vi "Auto Near Switch.vi"(10 "Right?":bool) -> ()   [LabVIEW 2017]
uses:
  Auto switch direita.ctl
  LabVIEW_is_Under_Control.lib/Util/Unpack Gamepad/Button Cluster.ctl
  Team Code/Robot Global Data.vi
panel:
  in  "90_time_limit":dbl=1800.0
  in  "Time_limit_fwd_2":dbl=1500.0 format="%#_13g"
  in  "Time_Limit_fwd":dbl=4000.0 format="%#_13g"
  in  "Delay fwd 2":i32=10
  in  "DistanceAfterTurn":dbl=40.0
  in  "Delay Turn":i32=150
  in  "Turn":dbl=-90.0 format="%#_13g"
  in  "Time to wait (min 50ms)":dbl=50.0
  in  "Delay Fwd":i32=100
  in  "DistanceSwitch":dbl=400.0
  out "auto state":T1=enum."Girando"
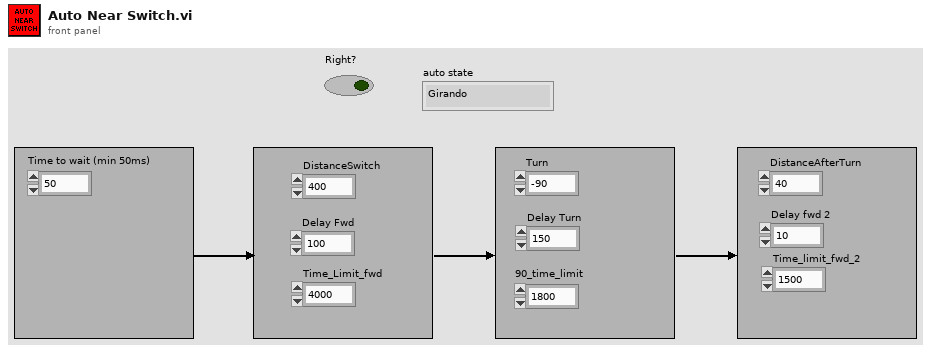
[diagram p1: front panel]
types:
  T1 = typedef "Auto switch direita.ctl" = enum16{"Zerandosensor", "Girando", "Andando", "Jogando", "Andando2", "Finalizando", "Zerandosensor2"}
  T2 = typedef "Button Cluster.ctl" = cluster{"Buttons[0]":bool, "Buttons[1]":bool, "Buttons[2]":bool, "Buttons[3]":bool, "Buttons[4]":bool, "Buttons[5]":bool, "Buttons[6]":bool, "Buttons[7]":bool, "Buttons[8]":bool, "Buttons[9]":bool}
  T3 = cluster{"proportional gain (Kc)":dbl, "integral time (Ti, min)":dbl, "derivative time (Td, min)":dbl}
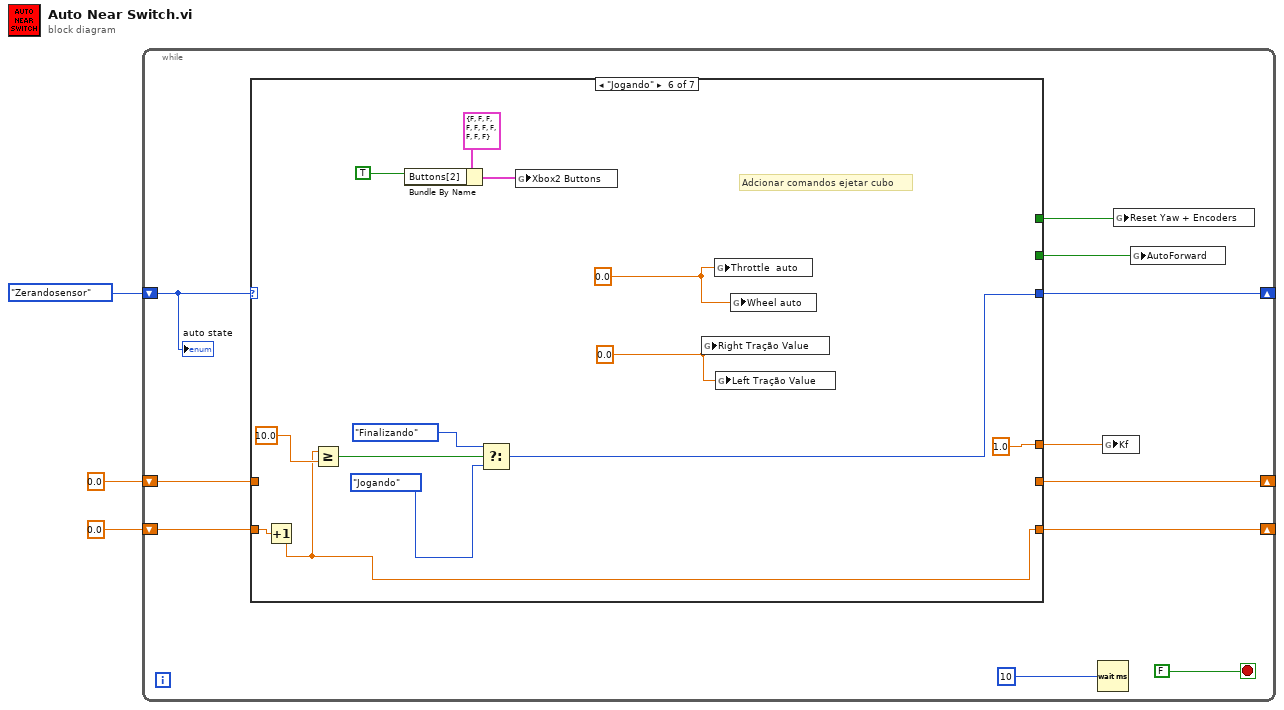
[diagram p0: block diagram]
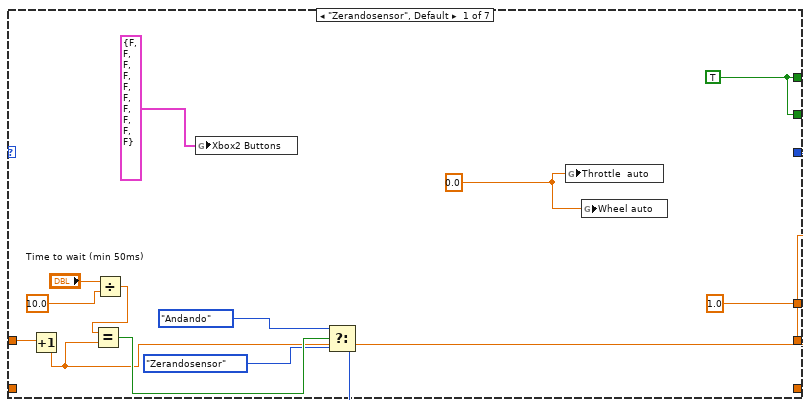
[diagram p2: hidden frame]
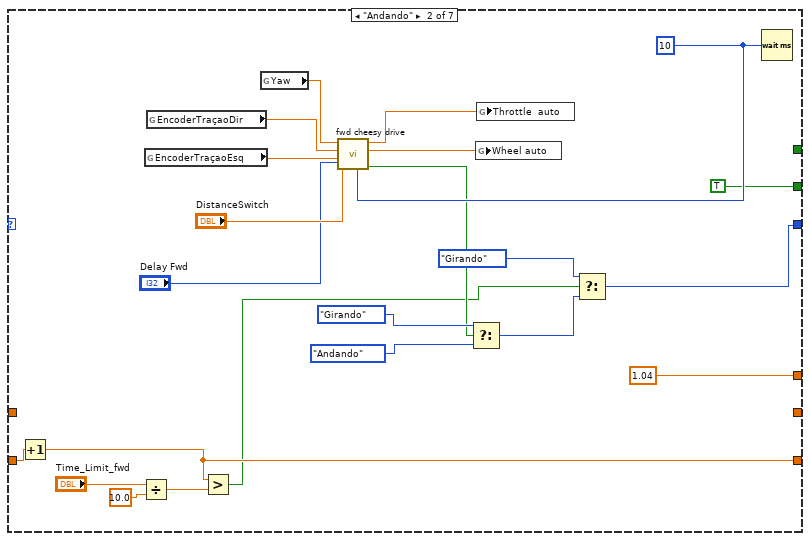
[diagram p3: hidden frame]
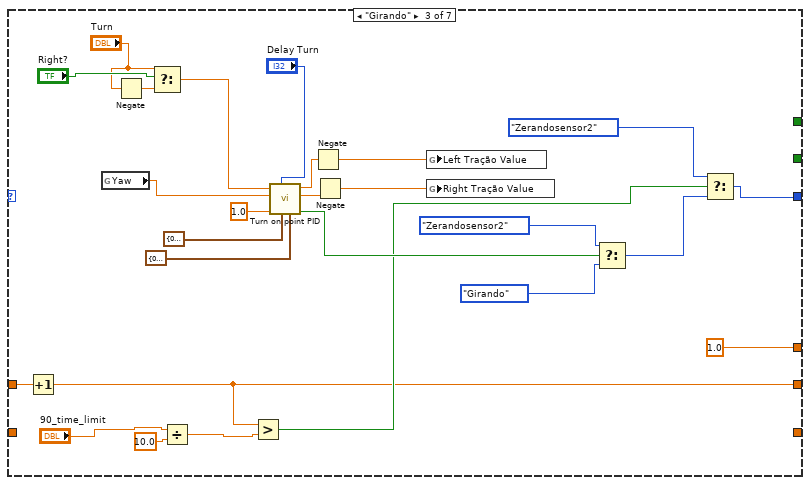
[diagram p4: hidden frame]
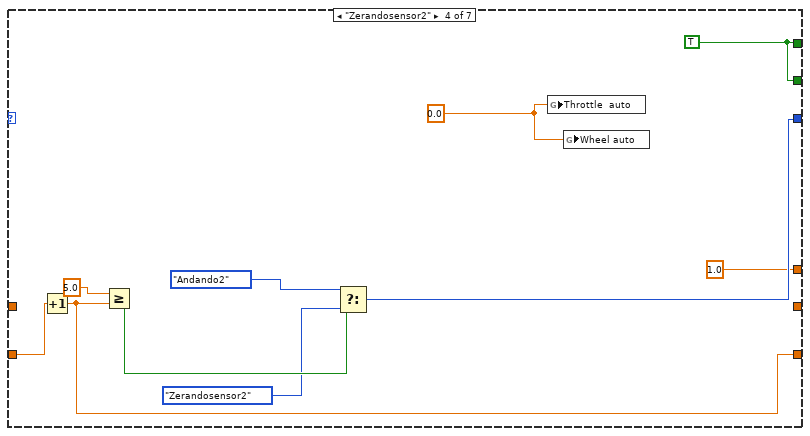
[diagram p5: hidden frame]
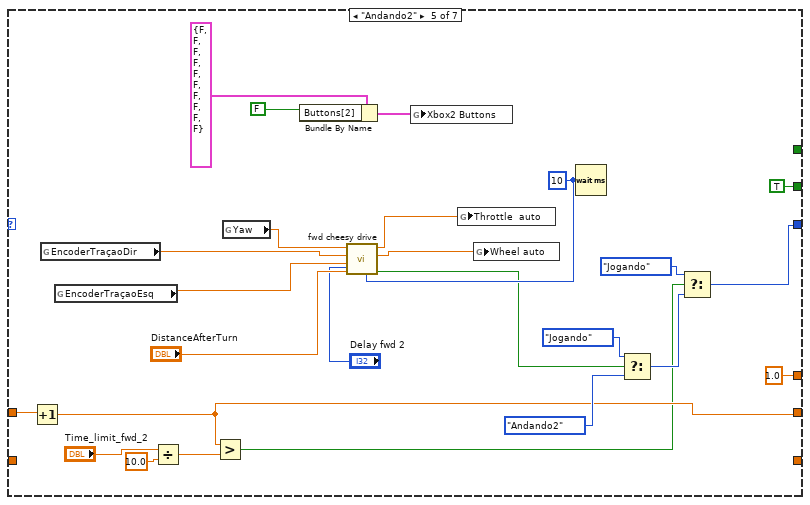
[diagram p6: hidden frame]
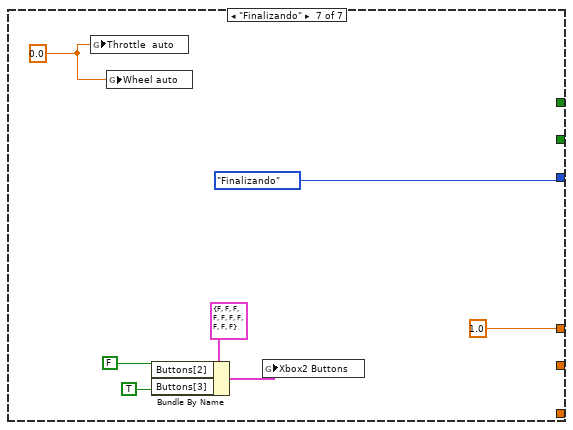
[diagram p7: hidden frame]
diagram:
  n1 = while {
    shift-right: [w10] -> _
    shift-left: Auto_switch_direita."Zerandosensor" -> [w8]
    shift-right: [w11] -> _
    shift-left: 0.0 -> [w12]
    shift-right: [w4] -> _
    shift-left: 0.0 -> [w5]
    stop <- FALSE stop-if-true
    n2 = case shown="\"Jogando\"" w8 {
      tunnel: w12 -> [w16 _ w53 _ w96 _ _]
      tunnel: [w26 _ w52 _ w95 _ _] -> w11
      tunnel: [w25 w35 w55 w79 w91 w122 Auto_switch_direita."Finalizando"] -> w10
      tunnel: [w22 _ _ w84 _ _ _] -> w7
      tunnel: [w22 TRUE _ w84 TRUE _ _] -> w9
      tunnel: [1.0 1.04 1.0 1.0 1.0 1.0 1.0] -> w6
      tunnel: w5 -> [_ w31 _ w77 _ w118 _]
      tunnel: [_ w30 _ w76 _ w111 _] -> w4
      frame "Zerandosensor", Default {
        w21 = 0.0
        w22 = TRUE
        n3 = Increment(x=w16) -> (x+1=w26:dbl)
        n4 = Divide(x="Time to wait (min 50ms)", y=10.0) -> (x/y=w17:dbl)
        n5 = Equal?(x=w17, y=w26) -> (x = y?=w27:bool)
        n6 = global write "Robot Global Data.vi" "Xbox2 Buttons"(T2 {"Buttons[0]"=FALSE, "Buttons[1]"=FALSE, "Buttons[2]"=FALSE, "Buttons[3]"=FALSE, "Buttons[4]"=FALSE, "Buttons[5]"=FALSE, "Buttons[6]"=FALSE, "Buttons[7]"=FALSE, "Buttons[8]"=FALSE, "Buttons[9]"=FALSE} ("Madcatz Buttons")) -> ()
        n7 = Select(t=Auto_switch_direita."Andando", s=w27, f=Auto_switch_direita."Zerandosensor") -> (s? t:f=w25:T1)
        n8 = global write "Robot Global Data.vi" "Throttle  auto"(w21) -> ()
        n9 = global write "Robot Global Data.vi" "Wheel auto"(w21) -> ()
      }
      frame "Andando" {
        w45 = u32 10 ("milliseconds to wait")
        n10 = Increment(x=w31) -> (x+1=w30:dbl)
        n11 = Divide(x="Time_Limit_fwd", y=10.0) -> (x/y=w32:dbl)
        n12 = global read "Robot Global Data.vi" "EncoderTraçaoEsq"() -> (w48:dbl)
        n13 = global read "Robot Global Data.vi" "EncoderTraçaoDir"() -> (w47:dbl)
        n14 = Greater?(x=w30, y=w32) -> (0:w28:bool)
        n15 = global read "Robot Global Data.vi" "Yaw"() -> (w49:dbl)
        n16 = call "fwd cheesy drive.vi"("Loop Timer"=w45, "Time to stop"="Delay Fwd", "Distance"="DistanceSwitch", "Encoder Left"=w48, "Encoder Right"=w47, "Yaw"=w49) -> ("Finished distance"=w29:bool, "Direction"=w43:dbl, "Trottle"=w42:dbl)  [unwired: 2 in, 1 out]
        n17 = Select(t=Auto_switch_direita."Girando", s=w29, f=Auto_switch_direita."Andando") -> (s? t:f=w36:T1)
        n18 = global write "Robot Global Data.vi" "Wheel auto"(w43) -> ()
        n19 = global write "Robot Global Data.vi" "Throttle  auto"(w42) -> ()
        n20 = Select(t=Auto_switch_direita."Girando", s=w28, f=w36) -> (s? t:f=w35:T1)
        n21 = Wait (ms)(milliseconds to wait=w45) -> ()  [unwired: 1 out]
      }
      frame "Girando" {
        n22 = Increment(x=w53) -> (x+1=w52:dbl)
        n23 = global read "Robot Global Data.vi" "Yaw"() -> (w68:dbl)
        n24 = Negate(x="Turn") -> (-x=w63:dbl)
        n25 = Select(t="Turn", s="Right?", f=w63) -> (s? t:f=w61:dbl)
        n26 = Divide(x="90_time_limit", y=10.0) -> (x/y=w59:dbl)
        n27 = Greater?(x=w52, y=w59) -> (0:w57:bool)
        n28 = call "Turn on point PID.vi"("Range"=cluster{"output high":dbl, "output low":dbl} {"output high"=0.65, "output low"=-0.65}, "Gains"=T3 {"proportional gain (Kc)"=0.015, "integral time (Ti, min)"=0.01, "derivative time (Td, min)"=0.0}, "Time to stop"="Delay Turn", "Precision"=1.0, "Yaw"=w68, "Setpoint(degrees)"=w61) -> ("Finished?"=w74:bool, "PWM right"=w70:dbl, "PWM left"=w71:dbl)  [unwired: 3 in]
        n29 = Negate(x=w71) -> (-x=w67:dbl)
        n30 = Negate(x=w70) -> (-x=w66:dbl)
        n31 = global write "Robot Global Data.vi" "Left Tração Value"(w67) -> ()
        n32 = global write "Robot Global Data.vi" "Right Tração Value"(w66) -> ()
        n33 = Select(t=Auto_switch_direita."Zerandosensor2", s=w74, f=Auto_switch_direita."Girando") -> (s? t:f=w56:T1)
        n34 = Select(t=Auto_switch_direita."Zerandosensor2", s=w57, f=w56) -> (s? t:f=w55:T1)
      }
      frame "Zerandosensor2" {
        w84 = TRUE
        w85 = 0.0
        n35 = Increment(x=w77) -> (x+1=w76:dbl)
        n36 = Greater Or Equal?(x=5.0, y=w76) -> (x >= y?=w82:bool)
        n37 = Select(t=Auto_switch_direita."Andando2", s=w82, f=Auto_switch_direita."Zerandosensor2") -> (s? t:f=w79:T1)
        n38 = global write "Robot Global Data.vi" "Throttle  auto"(w85) -> ()
        n39 = global write "Robot Global Data.vi" "Wheel auto"(w85) -> ()
      }
      frame "Andando2" {
        w107 = u32 10 ("milliseconds to wait")
        n40 = Increment(x=w96) -> (x+1=w95:dbl)
        n41 = global read "Robot Global Data.vi" "EncoderTraçaoDir"() -> (w89:dbl)
        n42 = global read "Robot Global Data.vi" "EncoderTraçaoEsq"() -> (w109:dbl)
        n43 = Divide(x="Time_limit_fwd_2", y=10.0) -> (x/y=w97:dbl)
        n44 = Greater?(x=w95, y=w97) -> (0:w93:bool)
        n45 = global read "Robot Global Data.vi" "Yaw"() -> (w110:dbl)
        n46 = Bundle By Name(cluster=T2 {"Buttons[0]"=FALSE, "Buttons[1]"=FALSE, "Buttons[2]"=FALSE, "Buttons[3]"=FALSE, "Buttons[4]"=FALSE, "Buttons[5]"=FALSE, "Buttons[6]"=FALSE, "Buttons[7]"=FALSE, "Buttons[8]"=FALSE, "Buttons[9]"=FALSE} ("Xbox Buttons"), "Buttons[2]"=FALSE) -> (w87:T2)
        n47 = call "fwd cheesy drive.vi"("Loop Timer"=w107, "Time to stop"="Delay fwd 2", "Distance"="DistanceAfterTurn", "Encoder Left"=w109, "Encoder Right"=w89, "Yaw"=w110) -> ("Finished distance"=w90:bool, "Direction"=w105:dbl, "Trottle"=w104:dbl)  [unwired: 2 in, 1 out]
        n48 = global write "Robot Global Data.vi" "Xbox2 Buttons"(w87) -> ()
        n49 = global write "Robot Global Data.vi" "Throttle  auto"(w104) -> ()
        n50 = global write "Robot Global Data.vi" "Wheel auto"(w105) -> ()
        n51 = Wait (ms)(milliseconds to wait=w107) -> ()  [unwired: 1 out]
        n52 = Select(t=Auto_switch_direita."Jogando", s=w90, f=Auto_switch_direita."Andando2") -> (s? t:f=w94:T1)
        n53 = Select(t=Auto_switch_direita."Jogando", s=w93, f=w94) -> (s? t:f=w91:T1)
      }
      frame "Jogando" {
        w116 = 0.0
        w117 = 0.0
        # "Adcionar comandos ejetar cubo"
        n54 = Increment(x=w118) -> (x+1=w111:dbl)
        n55 = Greater Or Equal?(x=w111, y=10.0) -> (x >= y?=w123:bool)
        n56 = Bundle By Name(cluster=T2 {"Buttons[0]"=FALSE, "Buttons[1]"=FALSE, "Buttons[2]"=FALSE, "Buttons[3]"=FALSE, "Buttons[4]"=FALSE, "Buttons[5]"=FALSE, "Buttons[6]"=FALSE, "Buttons[7]"=FALSE, "Buttons[8]"=FALSE, "Buttons[9]"=FALSE} ("Xbox Buttons"), "Buttons[2]"=TRUE) -> (w114:T2)
        n57 = Select(t=Auto_switch_direita."Finalizando", s=w123, f=Auto_switch_direita."Jogando") -> (s? t:f=w122:T1)
        n58 = global write "Robot Global Data.vi" "Xbox2 Buttons"(w114) -> ()
        n59 = global write "Robot Global Data.vi" "Right Tração Value"(w116) -> ()
        n60 = global write "Robot Global Data.vi" "Throttle  auto"(w117) -> ()
        n61 = global write "Robot Global Data.vi" "Left Tração Value"(w116) -> ()
        n62 = global write "Robot Global Data.vi" "Wheel auto"(w117) -> ()
      }
      frame "Finalizando" {
        w128 = 0.0
        n63 = global write "Robot Global Data.vi" "Throttle  auto"(w128) -> ()
        n64 = global write "Robot Global Data.vi" "Wheel auto"(w128) -> ()
        n65 = Bundle By Name(cluster=T2 {"Buttons[0]"=FALSE, "Buttons[1]"=FALSE, "Buttons[2]"=FALSE, "Buttons[3]"=FALSE, "Buttons[4]"=FALSE, "Buttons[5]"=FALSE, "Buttons[6]"=FALSE, "Buttons[7]"=FALSE, "Buttons[8]"=FALSE, "Buttons[9]"=FALSE} ("Xbox Buttons"), "Buttons[2]"=FALSE, "Buttons[3]"=TRUE) -> (w126:T2)
        n66 = global write "Robot Global Data.vi" "Xbox2 Buttons"(w126) -> ()
      }
    }
    n67 = Wait (ms)(milliseconds to wait=u32 10) -> ()  [unwired: 1 out]
    n68 = global write "Robot Global Data.vi" "Kf"(w6) -> ()
    n69 = global write "Robot Global Data.vi" "Reset Yaw + Encoders"(w7) -> ()
    n70 = global write "Robot Global Data.vi" "AutoForward"(w9) -> ()
    "auto state" <- w8
  }
